vi "Low Level Test.vi"() -> ()   [LabVIEW 2017]
uses:
  C:/Users/phorn/Documents/LV_SSH/Renci.SshNet.dll
  Renci.SshNet.dll
  ccbc5a90-95c6-4768-a4a1-e8d3a0ef45a0.vi
panel:
  out "Output Loop Count":i32
  out "UI Handler Loop Count":i32
  out "Output":string
  in  "value":string="exit"
  out "error out":errorcluster
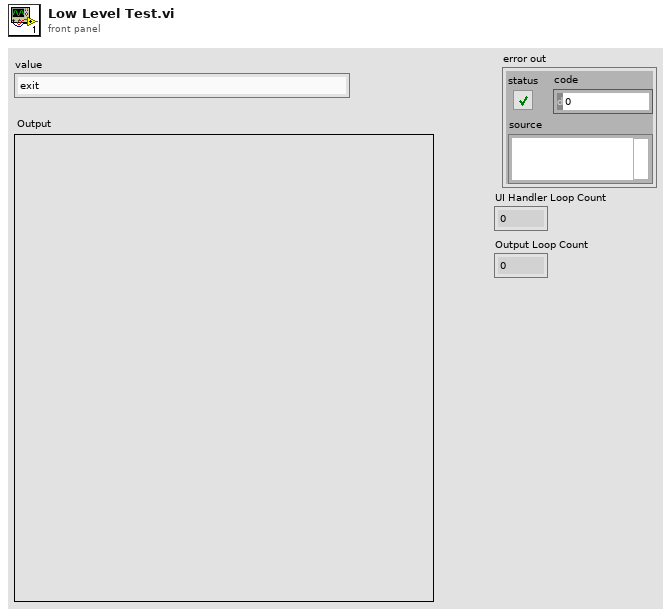
[diagram p1: front panel]
types:
  T1 = typedef "eventvkey.ctl" = enum16{"ASCII", "Enter", "Return", "Shift", "Ctrl", "Alt", "Cmd", "Opt", "Caps", "NumLock", "Clear", "Break", "Up", "Down", "Left", "Right", "Insert", "Delete", "Home", "End", "PageUp", "PageDown", "Escape", "Help", "Pause", "ScrollLock", "F1", "F2", "F3", "F4", "F5", "F6", "F7", "F8", "F9", "F10", "F11", "F12", "F13", "F14", "F15", "F16", "F17", "F18", "F19", "F20", "F21", "F22", "F23", "F24", "Play", "VolumeUp", "VolumeDown", "Mute", "Two Byte Char"}
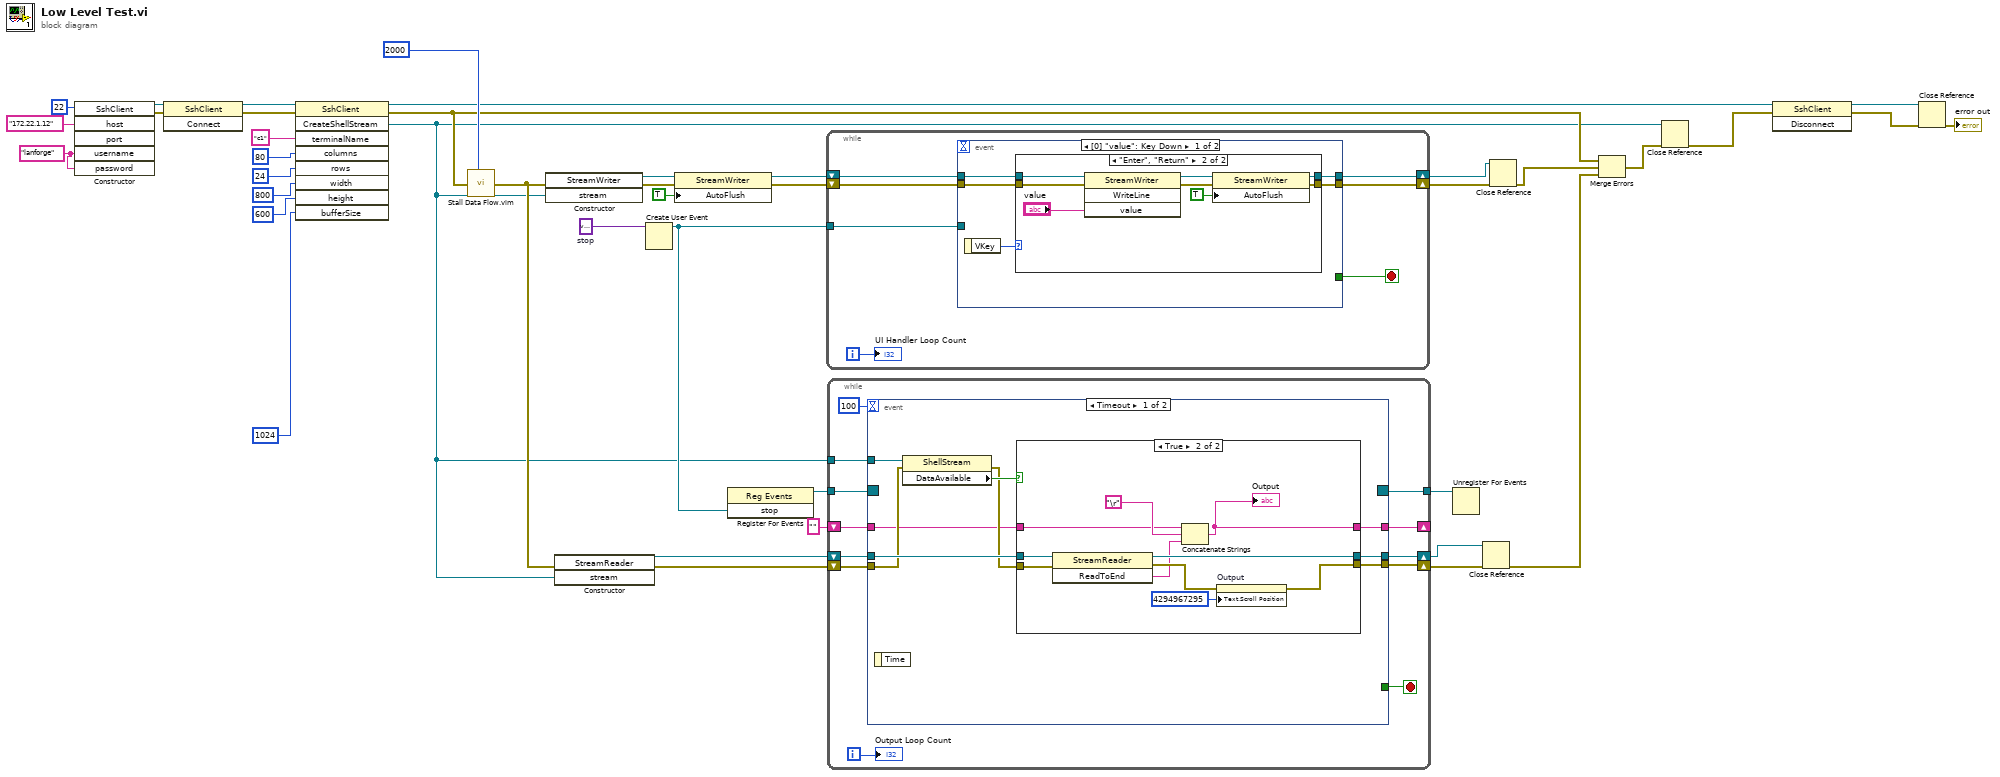
[diagram p0: block diagram]
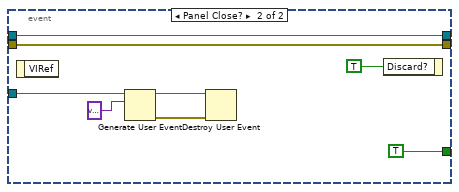
[diagram p3: hidden frame]
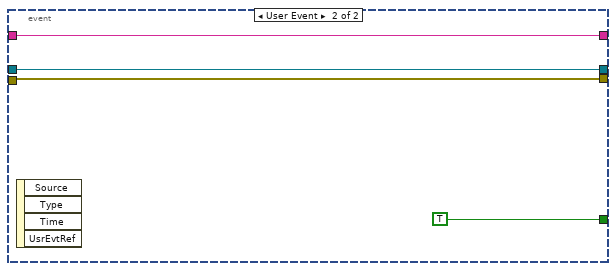
[diagram p5: hidden frame]
diagram:
  w18 = variant  # stop
  w2 = "lanforge" ("username")
  n1 = constructor class="SshClient"("host"="172.22.1.12", "port"=22, "username"=w2, "password"=w2) -> (reference out=w40:refnum<k24>, error out=w39:errorcluster)  [unwired: 3 in, 5 out]
  n2 = invoke class="SshClient" method="Connect"(reference=w40, error in=w39) -> (reference out=w38:refnum<k24>, error out=w37:errorcluster)  [unwired: 1 in, 1 out]
  n3 = invoke class="SshClient" method="CreateShellStream"(reference=w38, error in=w37, "terminalName"="c1", "columns"=u32 80, "rows"=u32 24, "width"=u32 800, "height"=u32 600, "bufferSize"=1024) -> (reference out=w4:refnum<k24>, error out=w10:errorcluster, "CreateShellStream"=w6:refnum<k24>)  [unwired: 1 in, 6 out]
  n4 = call "Stall Data Flow.vim"("value in"=w10, "milliseconds to wait"=u32 2000) -> ("value out"=w19:errorcluster)  [unwired: 1 out]
  n5 = constructor class="StreamWriter"(error in=w19, "stream"=w6) -> (reference out=w30:refnum<k24>, error out=w29:errorcluster)  [unwired: 2 in, 2 out]
  n6 = constructor class="StreamReader"(error in=w19, "stream"=w6) -> (reference out=w21:refnum<k24>, error out=w20:errorcluster)  [unwired: 2 in, 2 out]
  n7 = Create User Event(user event datatype=w18) -> (user event=w15:refnum<user-event>)  [unwired: 1 in, 1 out]
  n8 = property class="StreamWriter"(reference=w30, error in=w29, "AutoFlush"=TRUE) -> (reference out=w27:refnum<k24>, error out=w26:errorcluster)
  n9 = register-events(w15) -> (reference out=w17:refnum<event-registration>)  [unwired: 2 in, 1 out]
  n10 = while {
    shift-right: [w46] -> w25
    shift-left: w27 -> [w48]
    shift-right: [w45] -> w24
    shift-left: w26 -> [w47]
    tunnel: w15 -> [w44]
    i -> [w42]
    stop <- w43 stop-if-true
    n11 = event shown="[0] \"value\": Key Down" {
      selector: _ -> [_ _]
      dyn-events: _ -> [_ _]
      timeout: _ -> [_ _]
      tunnel: w48 -> [w53 w66]
      tunnel: w47 -> [w52 w65]
      tunnel: [w51 w66] -> w46
      tunnel: [w50 w65] -> w45
      tunnel: w44 -> [_ w68]
      tunnel: [_ TRUE ("Discard?")] -> w43
      event "value": Key Down {
        n12 = event-data() -> ("VKey"=w49:T1)  [unwired: 1 in]
        n13 = case shown="\"Enter\", \"Return\"" w49 {
          tunnel: w53 -> [w55 w62]
          tunnel: w52 -> [w54 w61]
          tunnel: [w55 w57] -> w51
          tunnel: [w54 w56] -> w50
          frame Default {
          }
          frame "Enter", "Return" {
            n14 = invoke class="StreamWriter" method="WriteLine"(reference=w62, error in=w61, "value"="value") -> (reference out=w60:refnum<k24>, error out=w59:errorcluster)  [unwired: 1 in, 2 out]
            n15 = property class="StreamWriter"(reference=w60, error in=w59, "AutoFlush"=TRUE) -> (reference out=w57:refnum<k24>, error out=w56:errorcluster)
          }
        }
      }
      event Panel Close? {
        n16 = event-data() -> ()  [unwired: 1 in, 1 out]
        n17 = Generate User Event(user event=w68, event data cluster=variant ("event data")) -> (user event out=w70:refnum<user-event>, error out=w69:errorcluster)  [unwired: 2 in]
        n18 = Destroy User Event(user event=w70, error in=w69) -> ()  [unwired: 1 out]
        n19 = event-data("Discard?"=TRUE) -> ()  [unwired: 1 in, 1 out]
      }
    }
    "UI Handler Loop Count" <- w42
  }
  n20 = while {
    tunnel: w6 -> [w83]
    tunnel: w17 -> [w79]
    tunnel: [w78] -> w16
    shift-right: [w76] -> w14
    shift-left: w21 -> [w82]
    shift-right: [w77] -> w13
    shift-left: w20 -> [w81]
    shift-right: [w73] -> _
    shift-left: "" -> [w72]
    i -> [w74]
    stop <- w75 stop-if-true
    n21 = event shown="[0] Timeout" {
      selector: w79 -> [_ _]
      dyn-events: [_ _] -> w78
      timeout: 100 -> [_ _]
      tunnel: w83 -> [w92 _]
      tunnel: w82 -> [w90 w109]
      tunnel: w81 -> [w87 w108]
      tunnel: [w89 w108] -> w77
      tunnel: [w88 w109] -> w76
      tunnel: [_ TRUE] -> w75
      tunnel: [w85 w106] -> w73
      tunnel: w72 -> [w84 w106]
      event Timeout {
        n22 = event-data() -> ()  [unwired: 1 in, 1 out]
        n23 = property class="ShellStream"(reference=w92, error in=w87) -> (error out=w86:errorcluster, "DataAvailable"=w91:bool)  [unwired: 1 out]
        n24 = case shown="True" w91 {
          tunnel: w90 -> [w95 w105]
          tunnel: w86 -> [w94 w104]
          tunnel: [w94 w97] -> w89
          tunnel: [w95 w102] -> w88
          tunnel: [w93 w98] -> w85
          tunnel: w84 -> [w93 w99]
          frame False {
          }
          frame True {
            n25 = invoke class="StreamReader" method="ReadToEnd"(reference=w105, error in=w104) -> (reference out=w102:refnum<k24>, error out=w103:errorcluster, "ReadToEnd"=w101:string)  [unwired: 1 in]
            n26 = Concatenate Strings(w99, "\r", w101) -> (w98:string)
            "Output" <- w98
            n27 = property on="Output" class="Str"(error in=w103, "Text.Scroll Position"=u32 4294967295) -> (error out=w97:errorcluster)  [unwired: 1 in, 1 out]
          }
        }
      }
      event User Event {
        n28 = event-data() -> ()  [unwired: 1 in, 4 out]
      }
    }
    "Output Loop Count" <- w74
  }
  n29 = Unregister For Events(event registration refnum=w16) -> ()  [unwired: 1 in, 1 out]
  n30 = Close Reference(reference=w14, error in (no error)=w13) -> (error out=w12:errorcluster)
  n31 = Close Reference(reference=w25, error in (no error)=w24) -> (error out=w11:errorcluster)
  n32 = Merge Errors(w10, w11, w12) -> (w9:errorcluster)
  n33 = Close Reference(reference=w6, error in (no error)=w9) -> (error out=w7:errorcluster)
  n34 = invoke class="SshClient" method="Disconnect"(reference=w4, error in=w7) -> (reference out=w3:refnum<k24>, error out=w5:errorcluster)  [unwired: 1 in, 1 out]
  n35 = Close Reference(reference=w3, error in (no error)=w5) -> (error out=→"error out":errorcluster)
